vi "String_request.vi"(8 "error in (no error)":errorcluster, 10 "SQL request":string, 11 "DB_SQLite in":refnum<class "DB_SQLite.lvclass">) -> (0 "error out":errorcluster, 2 "Result":string, 3 "DB_SQLite out":refnum<class "DB_SQLite.lvclass">)   [LabVIEW 2015, in "DB_SQLite.lvclass"]
uses:
  DB_SQLite.lvclass
  <vilib>/drjdpowell/SQLite Library/SQL Connection/Execute SQL (Single String).vi
  <vilib>/drjdpowell/SQLite Library/SQLite.lvlib
  <vilib>/drjdpowell/SQLite Library/SQL Connection/Connection.lvclass
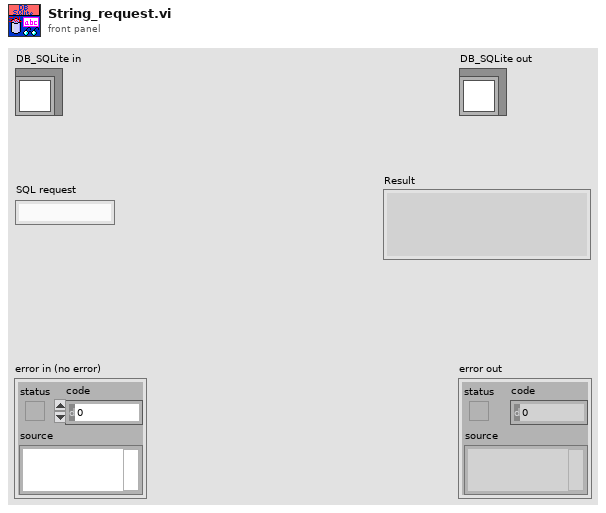
[diagram p1: front panel]
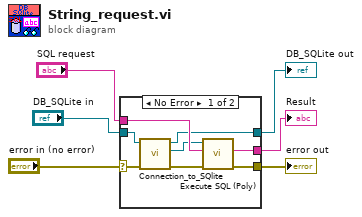
[diagram p0: block diagram]
diagram:
  n1 = case shown="No Error" "error in (no error)" {
    selector: "error in (no error)" -> [w12 w16]
    tunnel: [w14 _] -> w5
    tunnel: "SQL request" -> [w13 _]
    tunnel: [w10 w16] -> w3
    tunnel: "DB_SQLite in" -> [w7 w15]
    tunnel: [w8 w15] -> w1
    frame No Error {
      n2 = call "Connection_to_SQlite.vi"("error in (no error)"=w12, "DB_SQLite in"=w7) -> ("error out"=w11:errorcluster, "SQlite connection"=w9:refnum<class "Connection.lvclass">, "DB_SQLite out"=w8:refnum<class "DB_SQLite.lvclass">)  [unwired: 7 in]
      n3 = call-poly <vilib>:"Execute SQL (Poly).vi"("error in (no error)"=w11, "SQL"=w13, "SQLite Connection in"=w9) -> ("error out"=w10:errorcluster, "Result"=w14:string)  [unwired: 6 in, 1 out]
    }
    frame Error {
    }
  }
  "error out" <- w3
  "DB_SQLite out" <- w1
  "Result" <- w5
